vi "New Rx FIFO.vi"(8 "error in (no error)":errorcluster, 11 "Channel Number":u32) -> (0 "error out":errorcluster, 3 "Rx FIFO":refnum<k33>)   [LabVIEW 2020, in "985x Support Addon Engine.lvlib"]
uses:
  985x Support Addon Engine.lvlib
  985x Properties.vi
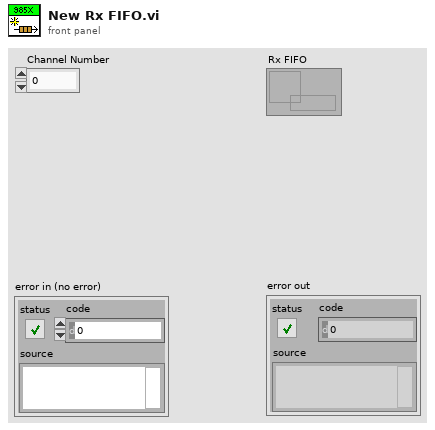
[diagram p1: front panel]
types:
  T1 = cluster{"read mode":enum16{"polling", "blocking"}, "write mode":enum16{"polling", "blocking"}}
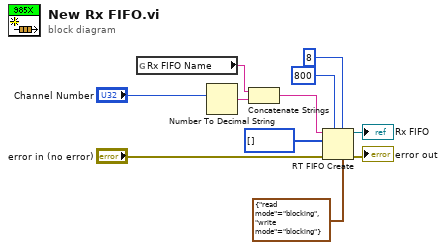
[diagram p0: block diagram]
diagram:
  n1 = global read "985x Properties.vi" "Rx FIFO Name"() -> (w11:string)
  n2 = Number To Decimal String(number="Channel Number") -> (decimal integer string=w10:string)  [unwired: 1 in]
  n3 = Concatenate Strings(w11, w10) -> (w9:string)
  n4 = RT FIFO Create(0:w9, 1:u32[] [], 3:"error in (no error)", 4:u32 800 ("size (10)"), 6:u32 8 ("elements in array (1)"), 7:T1 {"read mode"=enum."blocking", "write mode"=enum."blocking"} ("r/w modes (polling,polling)")) -> (8:→"Rx FIFO":refnum<k33>, 11:→"error out":errorcluster)  [unwired: 2 in, 1 out]
